vi "RGB565 to RGB.vi"(8 "error in (no error)":errorcluster, 10 "Color":u16, 11 "Color in":refnum<class "Color.lvclass">) -> (0 "error out":errorcluster, 3 "Color out":refnum<class "Color.lvclass">)   [LabVIEW 2020, in "RPI.SenseHat.Display.lvlib" / "Color.lvclass"]
doc: "Converts the RGB888 to the RGB565 color."
uses:
  Color.lvclass
  Color.lvclass/Color.ctl
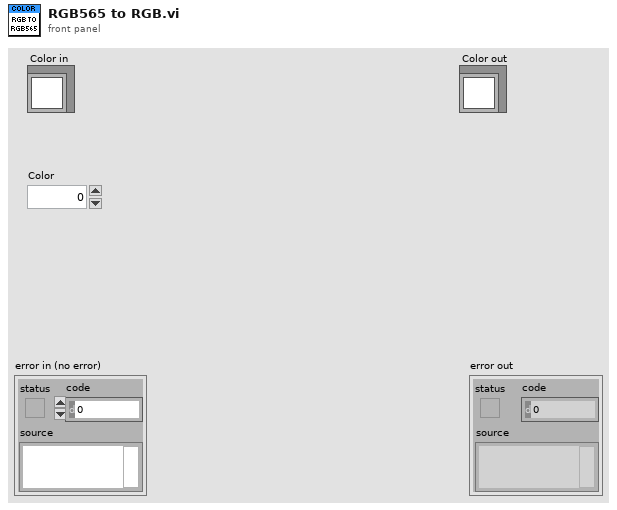
[diagram p1: front panel]
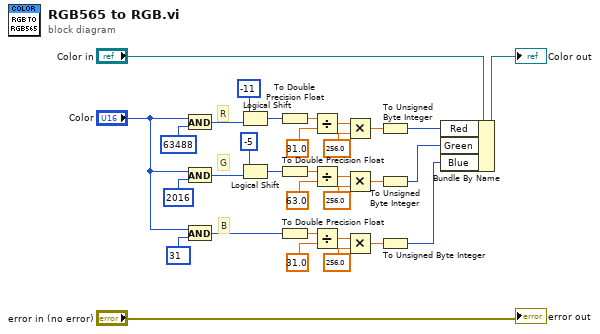
[diagram p0: block diagram]
diagram:
  # "B"
  # "G"
  # "R"
  n1 = And(x="Color", y=u16 63488) -> (x .and. y?=w13:u16)
  n2 = And(x="Color", y=u16 2016) -> (x .and. y?=w10:u16)
  n3 = And(x="Color", y=u16 31) -> (x .and. y?=w15:u16)
  n4 = Logical Shift(y=i16 -11, x=w13) -> (x << y=w14:u16)
  n5 = Logical Shift(y=i16 -5, x=w10) -> (x << y=w11:u16)
  n6 = To Double Precision Float(number=w14) -> (double precision float=w30:dbl)
  n7 = To Double Precision Float(number=w11) -> (double precision float=w21:dbl)
  n8 = To Double Precision Float(number=w15) -> (double precision float=w20:dbl)
  n9 = Divide(x=w30, y=31.0) -> (x/y=w29:dbl)
  n10 = Divide(x=w21, y=63.0) -> (x/y=w22:dbl)
  n11 = Divide(x=w20, y=31.0) -> (x/y=w19:dbl)
  n12 = Multiply(x=w29, y=256.0) -> (x*y=w27:dbl)
  n13 = Multiply(x=w22, y=256.0) -> (x*y=w24:dbl)
  n14 = Multiply(x=w19, y=256.0) -> (x*y=w17:dbl)
  n15 = To Unsigned Byte Integer(number=w27) -> (unsigned 8bit integer=w3:u8)
  n16 = To Unsigned Byte Integer(number=w24) -> (unsigned 8bit integer=w2:u8)
  n17 = To Unsigned Byte Integer(number=w17) -> (unsigned 8bit integer=w1:u8)
  n18 = Bundle By Name(cluster="Color in", "Red"=w3, "Green"=w2, "Blue"=w1) -> (→"Color out":refnum<class "Color.lvclass">)
  "error out" <- "error in (no error)"
